vi "DSF.Execution.Runtime.Plugin Manager.Set Plugins Folder.vi"(8 "error in (no error)":errorcluster, 10 "Plugins folder":path, 11 "Plugin Manager in":refnum<class "DSF.Engine.Runtime.Plugin Manager.lvclass">) -> (0 "error out":errorcluster, 3 "Plugin Manager out":refnum<class "DSF.Engine.Runtime.Plugin Manager.lvclass">)   [LabVIEW 2016, in "DSF.Engine.lvlib" / "DSF.Engine.Runtime.Plugin Manager.lvclass"]
uses:
  DSF.Engine.Runtime.Plugin Manager.lvclass
  DSF.Engine.Runtime.Plugin Manager.lvclass/DSF.Engine.Runtime.Plugin Manager.ctl
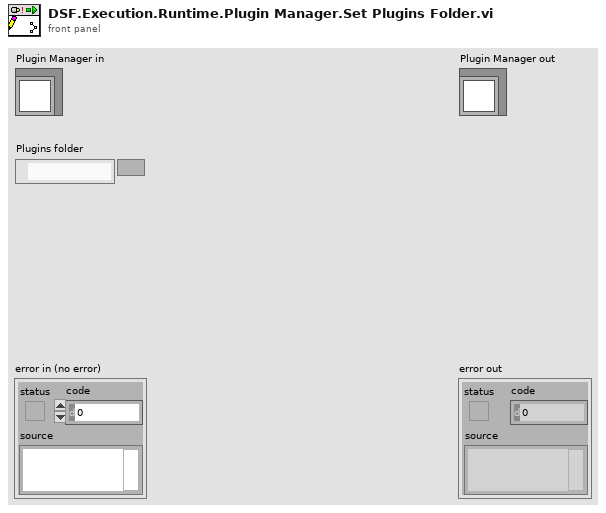
[diagram p1: front panel]
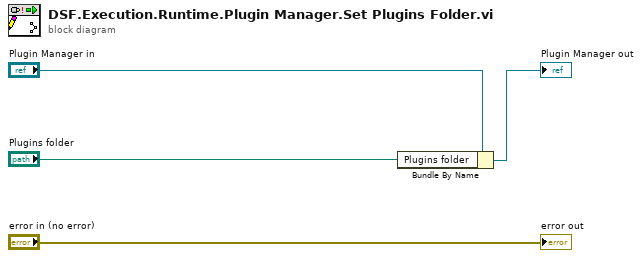
[diagram p0: block diagram]
diagram:
  n1 = Bundle By Name(cluster="Plugin Manager in", "Plugins folder"="Plugins folder") -> (→"Plugin Manager out":refnum<class "DSF.Engine.Runtime.Plugin Manager.lvclass">)
  "error out" <- "error in (no error)"
